vi "Clad practice-1.vi"() -> ()   [LabVIEW 2020]
panel:
  out "Waveform Graph 2":i32[](graph)
  out "Iteration's":i32[](array[numeric])
  out "Array":i32[](array[numeric])
  out "4":i32
  out "3":i32
  out "2":i32
  out "1":i32
  out "Waveform Graph":i32[](graph)
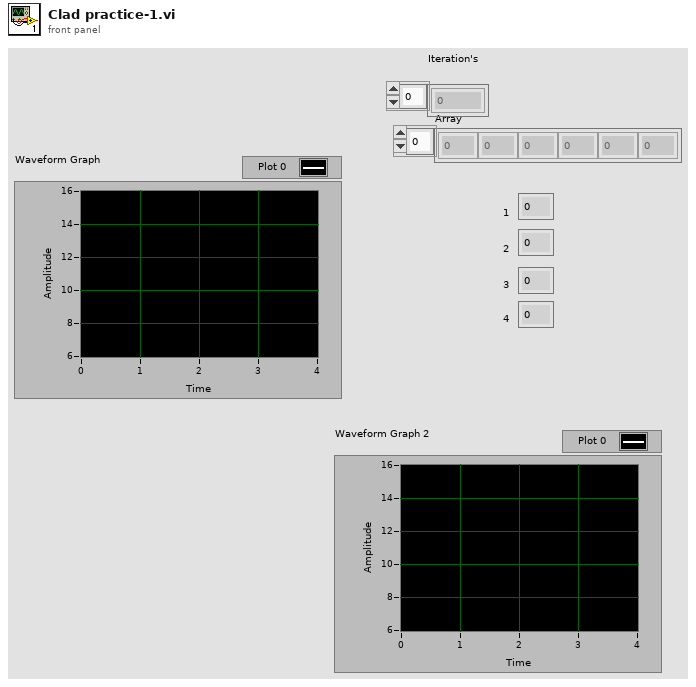
[diagram p1: front panel]
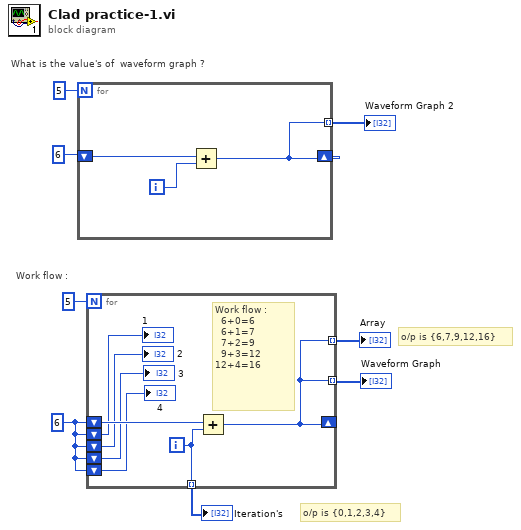
[diagram p0: block diagram]
diagram:
  w6 = 6
  # "Work flow :"
  # "o/p is {0,1,2,3,4}"
  # "What is the value's of  waveform graph ?"
  # "o/p is {6,7,9,12,16}"
  n1 = for {
    N: 5 -> [_]
    shift-right: [w9] -> _
    shift-left: 6 -> [w10]
    tunnel: [w9] -> w1 mode=indexing
    i -> [w11]
    n2 = Add(x=w10, y=w11) -> (x+y=w9:i32)
  }
  "Waveform Graph 2" <- w1
  n3 = for {
    N: 5 -> [_]
    shift-right: [w13] -> _
    shift-left: w6 -> [w18]
    tunnel: [w13] -> w7 mode=indexing
    shift-left: w6 -> [w17]
    shift-left: w6 -> [w14]
    shift-left: w6 -> [w15]
    shift-left: w6 -> [w16]
    tunnel: [w13] -> w5 mode=indexing
    tunnel: [w12] -> w4 mode=indexing
    i -> [w12]
    # "Work flow :  \n  6+0=6\n  6+1=7\n  7+2=9\n  9+3=12\n12+4=16"
    n4 = Add(x=w18, y=w12) -> (x+y=w13:i32)
    "1" <- w17
    "2" <- w14
    "4" <- w16
    "3" <- w15
  }
  "Waveform Graph" <- w7
  "Array" <- w5
  "Iteration's" <- w4
